vi "Motor drive.vi"(11 "RobotDriveDevRef":T1={"DevStatus"={"status"=FALSE, "code"=0, "source"=""}, "Motors[]"=[], "Square Inputs"=FALSE, "Max Output"=1.0}) -> (10 "Boolean":bool)   [LabVIEW 2014]
uses:
  <vilib>/Rock Robotics/WPI/RobotDrive/WPI_RobotDriveDevRef.ctl
  <vilib>/Rock Robotics/WPI/MotorControl/WPI_MotorControlDeviceRef.ctl
  <vilib>/Rock Robotics/SystemInterfaces/Typedef/FPGA_TypedefDigitalModule.ctl
  <vilib>/Rock Robotics/SystemInterfaces/DIO/FPGA_DIOPWMChannel.ctl
  <vilib>/Rock Robotics/WPI/PWM/WPI_PWMDeadband.ctl
  <vilib>/Rock Robotics/WPI/CAN/Jaguar/SubVIs/WPI_CANJaguar_ControlMode.ctl
  <vilib>/Rock Robotics/WPI/PWM/WPI_PWMTransform_ConPane.ctl
  <vilib>/Rock Robotics/WPI/DriverStation/WPI_DriverStationRobotMode2.ctl
  Events.vi
  Robot Global Data.vi
  <vilib>/Rock Robotics/WPI/RobotDrive/WPI_RobotDriveArcadeDrive_Standard(NoSaturation).vi
  <vilib>/Rock Robotics/WPI/RobotDrive/WPI_RobotDriveMecanumDrive_Cartesian.vi
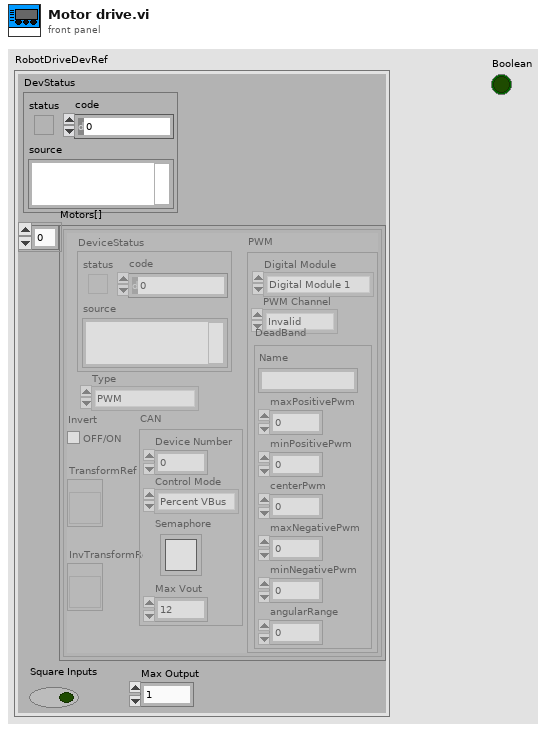
[diagram p1: front panel]
types:
  T1 = typedef "WPI_RobotDriveDevRef.ctl" = cluster{"DevStatus":errorcluster, "Motors[]":T2[], "Square Inputs":bool, "Max Output":dbl}
  T2 = typedef "WPI_MotorControlDeviceRef.ctl" = cluster{"DeviceStatus":errorcluster, "Type":enum16{"PWM", "CAN"}, "PWM":cluster{"Digital Module":T3, "PWM Channel":T4, "DeadBand":T5}, "CAN":cluster{"Device Number":u8, "Control Mode":T6, "Semaphore":T7, "Max Vout":dbl}, "Invert":bool, "TransformRef":T8, "InvTransformRef":T8}
  T3 = typedef "FPGA_TypedefDigitalModule.ctl" = enum16{"Digital Module 1", "Digital Module 2"}
  T4 = typedef "FPGA_DIOPWMChannel.ctl" = enum8{"PWM 1", "PWM 2", "PWM 3", "PWM 4", "PWM 5", "PWM 6", "PWM 7", "PWM 8", "PWM 9", "PWM 10", "Invalid"}
  T5 = typedef "WPI_PWMDeadband.ctl" = cluster{"Name":string, "maxPositivePwm":i32, "minPositivePwm":i32, "centerPwm":i32, "maxNegativePwm":i32, "minNegativePwm":i32, "angularRange":u16}
  T6 = typedef "WPI_CANJaguar_ControlMode.ctl" = enum8{"Percent VBus", "Current", "Speed", "Position", "Voltage"}
  T7 = typedef "Semaphore RefNum" = refnum<k1>
  T8 = typedef "WPI_PWMTransform_ConPane.ctl" = refnum<vi>
  T9 = typedef "WPI_DriverStationRobotMode2.ctl" = enum16{"Autonomous Disabled", "Autonomous Enabled", "Teleop Disabled", "Teleop Enabled", "Disconnected", "Finish", "Test Disabled", "Test Enabled"}
  T10 = cluster{"Translate":dbl, "Y-Axis (Backward Speed)":dbl, "Rotate":dbl, "Tank right side":dbl, "axis 5":dbl, "axis 6":dbl, "Use gyro":bool, "Exponential\ndrive":bool, "Ring light":bool, "PID rotation":bool, "PID Gain":dbl}
  T11 = typedef "WPI_SolenoidValue.ctl" = enum16{"Off", "On", "Forward", "Reverse"}
  T12 = cluster{"Ultrasonic Distance (In)":dbl, "Gyro":dbl, "TopAquisition sensor":bool, "Encoder distance":dbl, "Encoder rate":dbl, "Encoder direction":bool, "winch engaged?":T11, "Motor Values":dbl[], "Latch encoder":u32, "BottomAquistion":bool, "BottomAquistion 2":bool, "Gyro Rate":dbl}
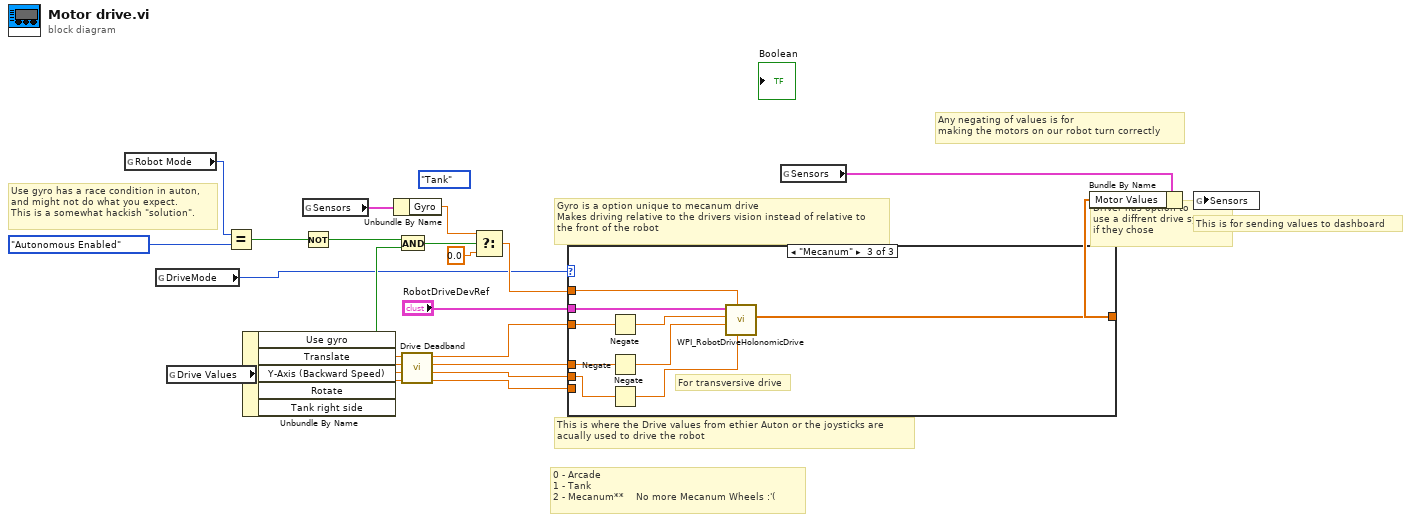
[diagram p0: block diagram]
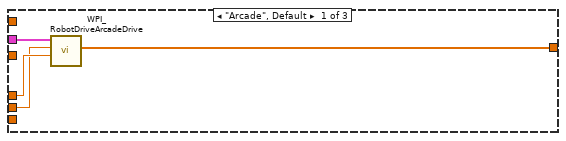
[diagram p2: hidden frame]
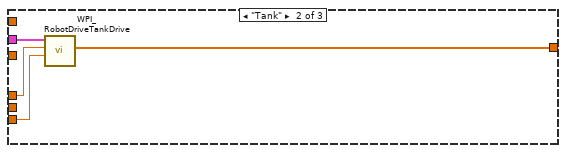
[diagram p3: hidden frame]
diagram:
  (unwired) enum16{"Arcade", "Mecanium", "Tank"}."Tank"
  # "0 - Arcade\n1 - Tank\n2 - Mecanum**    No more Mecanum Wheels :'("
  # "Use gyro has a race condition in auton,\nand might not do what you expect.\nThis is a somewhat hackish \"solution\"."
  # "This is for sending values to dashboard"
  # "Gyro is a option unique to mecanum drive\nMakes driving relative to the drivers vision instead of relative to\nthe front of the robot"
  # "Driver has option to\nuse a diffrent drive system\nif they chose"
  # "Any negating of values is for\nmaking the motors on our robot turn correctly"
  # "This is where the Drive values from ethier Auton or the joysticks are \nacually used to drive the robot"
  n1 = global read "Robot Global Data.vi" "Robot Mode"() -> (w16:T9)
  n2 = global read "Events.vi" "DriveMode"() -> (w1:enum16{"Arcade", "Tank", "Mecanum"})
  n3 = global read "Events.vi" "Drive Values"() -> (w23:T10)
  n4 = Equal?(x=w16, y=WPI_DriverStationRobotMode2."Autonomous Enabled") -> (x = y?=w14:bool)
  n5 = Unbundle By Name(w23) -> ("Use gyro"=w18:bool, "Translate"=w9:dbl, "Y-Axis (Backward Speed)"=w2:dbl, "Rotate"=w3:dbl, "Tank right side"=w4:dbl)
  n6 = global read "Events.vi" "Sensors"() -> (w22:T12)
  n7 = Not(x=w14) -> (.not. x?=w13:bool)
  n8 = Unbundle By Name(w22) -> ("Gyro"=w21:dbl)
  n9 = And(x=w13, y=w18) -> (x .and. y?=w17:bool)
  n10 = call "Drive Deadband.vi"("Tank"=w4, "Rotate"=w3, "Forward"=w2, "Translate"=w9) -> ("Tank"=w5:dbl, "Rotate"=w6:dbl, "Forward"=w7:dbl, "Translate"=w8:dbl)  [unwired: 4 in]
  n11 = Select(t=w21, s=w17, f=0.0) -> (s? t:f=w19:dbl)
  n12 = case shown="\"Mecanum\"" w1 {
    tunnel: "RobotDriveDevRef" -> [w28 w32 w41]
    tunnel: w8 -> [_ _ w40]
    tunnel: w7 -> [w27 w31 w39]
    tunnel: w6 -> [w26 _ w38]
    tunnel: w5 -> [_ w30 _]
    tunnel: w19 -> [_ _ w37]
    tunnel: [w25 w29 w33] -> w10
    frame "Arcade", Default {
      n13 = call-poly <vilib>:"WPI_RobotDriveArcadeDrive.vi"("Y axis value"=w27, "X axis value"=w26, "RobotDriveDevRef"=w28) -> ("Motor Values"=w25:dbl[])  [unwired: 6 in, 2 out]
    }
    frame "Tank" {
      n14 = call <vilib>:"WPI_RobotDriveTankDrive.vi"("Right axis value"=w30, "Left axis value"=w31, "RobotDriveDevRef"=w32) -> ("Motor Values"=w29:dbl[])  [unwired: 6 in, 2 out]
    }
    frame "Mecanum" {
      # "For transversive drive"
      n15 = Negate(x=w40) -> (-x=w34:dbl)
      n16 = Negate(x=w39) -> (-x=w36:dbl)
      n17 = Negate(x=w38) -> (-x=w35:dbl)
      n18 = call-poly <vilib>:"WPI_RobotDriveHolonomicDrive.vi"("Rotation"=w35, "Gyro Angle"=w37, "Y"=w36, "X"=w34, "RobotDriveDevRef"=w41) -> ("Motor Values"=w33:dbl[])  [unwired: 4 in, 2 out]
    }
  }
  n19 = global read "Events.vi" "Sensors"() -> (w11:T12)
  n20 = Bundle By Name(cluster=w11, "Motor Values"=w10) -> (w12:T12)
  n21 = global write "Events.vi" "Sensors"(w12) -> ()
